vi "Bode Magnitude Plot.vi"() -> ()   [LabVIEW 2015]
uses:
  <vilib>/Analysis/NI_AALPro.lvlib
panel:
  out "Frequency":dbl
  out "XY Graph":cluster{dbl[], dbl[]}(graph)
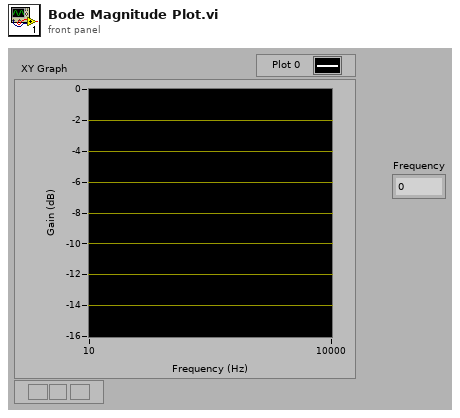
[diagram p1: front panel]
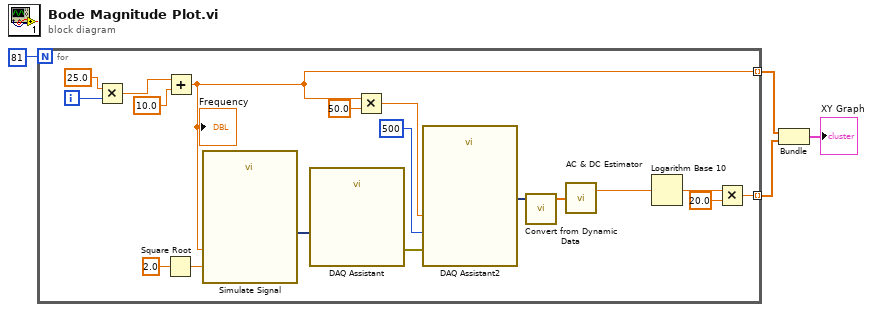
[diagram p0: block diagram]
diagram:
  n1 = for {
    N: 81 -> [_]
    tunnel: [w6] -> w2 mode=indexing
    tunnel: [w10] -> w3 mode=indexing
    i -> [w19]
    n2 = Multiply(x=25.0, y=w19) -> (x*y=w17:dbl)
    n3 = Square Root(x=2.0) -> (sqrt(x)=w21:dbl)
    n4 = Add(x=w17, y=10.0) -> (x+y=w10:dbl)
    "Frequency" <- w10
    n5 = call "Simulate Signal"("Frequency"=w10, "Amplitude"=w21) -> ("Sine"=w20:dynamicdata)  [unwired: 12 in, 1 out]
    n6 = call "DAQ Assistant"("data"=w20) -> ("error out"=w5:errorcluster)  [unwired: 16 in, 2 out]
    n7 = Multiply(x=w10, y=50.0) -> (x*y=w14:dbl)
    n8 = call "DAQ Assistant2"("rate"=w14, "number of samples"=500, "error in"=w5) -> ("data"=w12:dynamicdata)  [unwired: 14 in, 2 out]
    n9 = call "Convert from Dynamic Data"("Dynamic Data Type"=w12) -> ("Array"=w11:dbl[])  [unwired: 3 in]
    n10 = call <vilib>:"AC & DC Estimator.vi"("Signal (V)"=w11) -> ("AC estimate (Vrms)"=w9:dbl)  [unwired: 1 out]
    n11 = Logarithm Base 10(1:w9) -> (0:w8:dbl)
    n12 = Multiply(x=w8, y=20.0) -> (x*y=w6:dbl)
  }
  n13 = Bundle(w3, w2) -> (→"XY Graph":cluster{dbl[], dbl[]})  [unwired: 1 in]
